vi "Prepare Execution.vi"(0 "Session Handle in":T3, 2 "Options (Default)":T1={"Use Default Model"=FALSE, "Release Related Sessions"=TRUE}, 11 "error in (no error)":errorcluster) -> (4 "Session Handle out":T3, 8 "Execution":T2, 15 "error out":errorcluster)   [LabVIEW 2020, in "TSS.lvlib" / "Engine.lvclass"]
uses:
  Engine.lvclass
  Typedefs/Session Handle.ctl
  Execution/Typedefs/Session Handle.ctl
  Execution/Execution.lvclass
  Execution/Execution Options.ctl
  Session Notification.ctl
  Prepare Execution Event Data.ctl
  Engine.lvclass/Engine.ctl
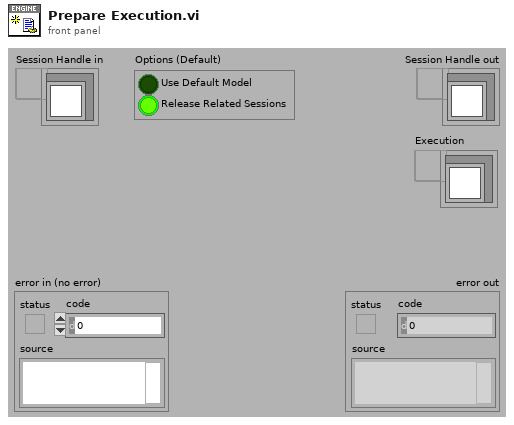
[diagram p1: front panel]
types:
  T1 = typedef "TSS.lvlib/Execution.lvclass/Execution Options.ctl" = cluster{"Use Default Model":bool, "Release Related Sessions":bool}
  T2 = typedef "TSS.lvlib/Execution.lvclass/Session Handle.ctl" = refnum<data-value>
  T3 = typedef "TSS.lvlib/Engine.lvclass/Session Handle.ctl" = refnum<data-value>
  T4 = typedef "TSS.lvlib/Engine.lvclass/Prepare Execution Event Data.ctl" = cluster{"Execution Options":T1, "Engine":refnum<data-value>, "Session Notifier":refnum<notifier>}
  T5 = typedef "TSS.lvlib/Engine.lvclass/Session Notification.ctl" = cluster{"Session":refnum<data-value>, "Error":errorcluster}
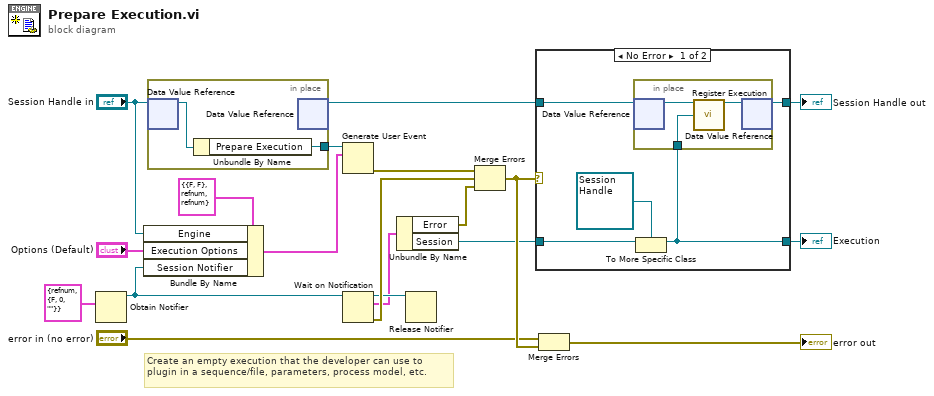
[diagram p0: block diagram]
diagram:
  # "Create an empty execution that the developer can use to plugin in a sequence/file, parameters, process model, etc."
  n1 = Obtain Notifier(notification data type=T5 {"Session"=refnum, "Error"={"status"=FALSE, "code"=0, "source"=""}} ("Session Notification")) -> (notifier out=w9:refnum<notifier>)  [unwired: 3 in, 2 out]
  n2 = Bundle By Name(cluster=T4 {"Execution Options"={"Use Default Model"=FALSE, "Release Related Sessions"=FALSE}, "Engine"=refnum, "Session Notifier"=refnum} ("Prepare Execution Event Data"), "Engine"="Session Handle in", "Execution Options"="Options (Default)", "Session Notifier"=w9) -> (w11:T4)
  n3 = in-place {
    in-place-border: [w20] -> w12
    n4 = in-place-dvr #1("Session Handle in") -> (w21:refnum<class "Engine.lvclass">)  [unwired: 1 out]
    n5 = Unbundle By Name(w21) -> ("Prepare Execution"=w20:refnum<user-event>)
    n6 = in-place-dvr #1() -> (w10:T3)  [unwired: 1 in, 1 out]
  }
  n7 = Generate User Event(user event=w12, event data cluster=w11) -> (error out=w7:errorcluster)  [unwired: 2 in, 1 out]
  n8 = Wait on Notification(notifier=w9) -> (notifier out=w8:refnum<notifier>, notification=w6:T5, error out=w19:errorcluster)  [unwired: 3 in, 1 out]
  n9 = Unbundle By Name(w6) -> ("Error"=w5:errorcluster, "Session"=w4:refnum<data-value>)
  n10 = Release Notifier(notifier=w8) -> ()  [unwired: 2 in, 3 out]
  n11 = Merge Errors(w7, w19, w5) -> (w18:errorcluster)
  n12 = case shown="No Error" w18 {
    tunnel: [w26 w30] -> w17
    tunnel: w10 -> [w25 w30]
    tunnel: w4 -> [w24 _]
    tunnel: [w22 _] -> w3
    frame No Error {
      n13 = To More Specific Class(target class=T2 refnum ("Execution"), reference=w24) -> (specific class reference=w22:T2)  [unwired: 1 in, 1 out]
      n14 = in-place {
        in-place-border: w22 -> [w27]
        n15 = in-place-dvr #2(w25) -> (w29:refnum<class "Engine.lvclass">)  [unwired: 1 out]
        n16 = call "Register Execution.vi"("Engine in"=w29, "Execution"=w27) -> ("Engine out"=w28:refnum<class "Engine.lvclass">)  [unwired: 12 in, 1 out]
        n17 = in-place-dvr #2(w28) -> (w26:T3)  [unwired: 1 out]
      }
    }
    frame Error {
    }
  }
  "Session Handle out" <- w17
  "Execution" <- w3
  n18 = Merge Errors("error in (no error)", w18) -> (→"error out":errorcluster)
